vi "Read Wait (ms).vi"(8 "error in (no error)":errorcluster, 11 "Wait Step in":refnum<class "Wait Step.lvclass">) -> (0 "error out":errorcluster, 2 "Wait (ms)":u32, 3 "Wait Step out":refnum<class "Wait Step.lvclass">)   [LabVIEW 2015, in "Wait Step.lvclass"]
uses:
  Wait Step.lvclass
  Wait Step.lvclass/Wait Step.ctl
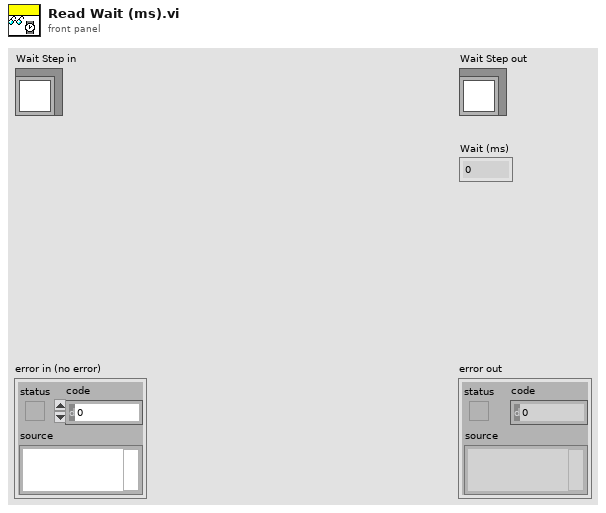
[diagram p1: front panel]
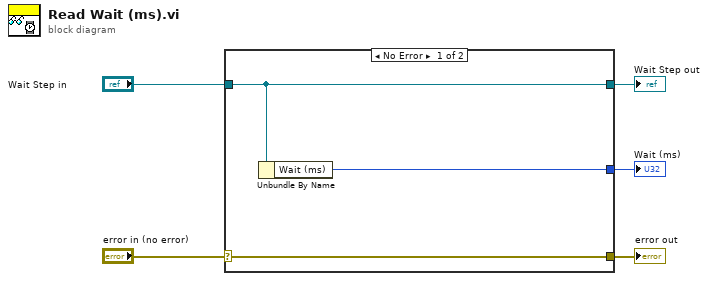
[diagram p0: block diagram]
diagram:
  n1 = case shown="No Error" "error in (no error)" {
    selector: "error in (no error)" -> [w8 w9]
    tunnel: [w8 w9] -> w4
    tunnel: [w7 w10] -> w2
    tunnel: "Wait Step in" -> [w7 w10]
    tunnel: [w6 _] -> w1
    frame No Error {
      n2 = Unbundle By Name(w7) -> ("Wait (ms)"=w6:u32)
    }
    frame Error {
    }
  }
  "error out" <- w4
  "Wait Step out" <- w2
  "Wait (ms)" <- w1
